vi "Read_fastseq.vi"(2 "Sequence size":u64, 5 "Readout parameters":T1(array[cluster])) -> (0 "measures":sgl[][](array[numeric]), 1 "Readout parameters out":T1(array[cluster]))   [LabVIEW 2013]
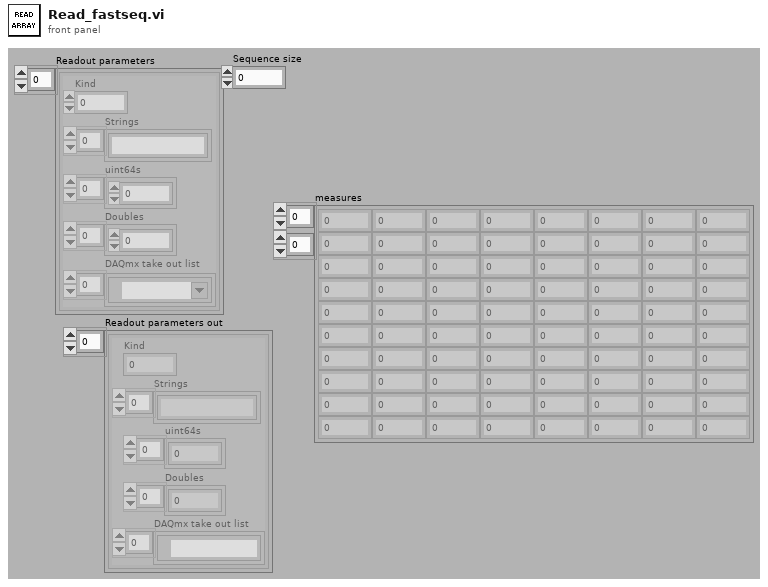
[diagram p1: front panel]
types:
  T1 = cluster{"Kind":u16, "Strings":string[], "uint64s":u64[], "Doubles":dbl[], "DAQmx take out list":refnum<k21>[]}[]
  T2 = cluster{"Kind":u16, "Strings":string[], "uint64s":u64[], "Doubles":dbl[], "DAQmx take out list":refnum<k21>[]}
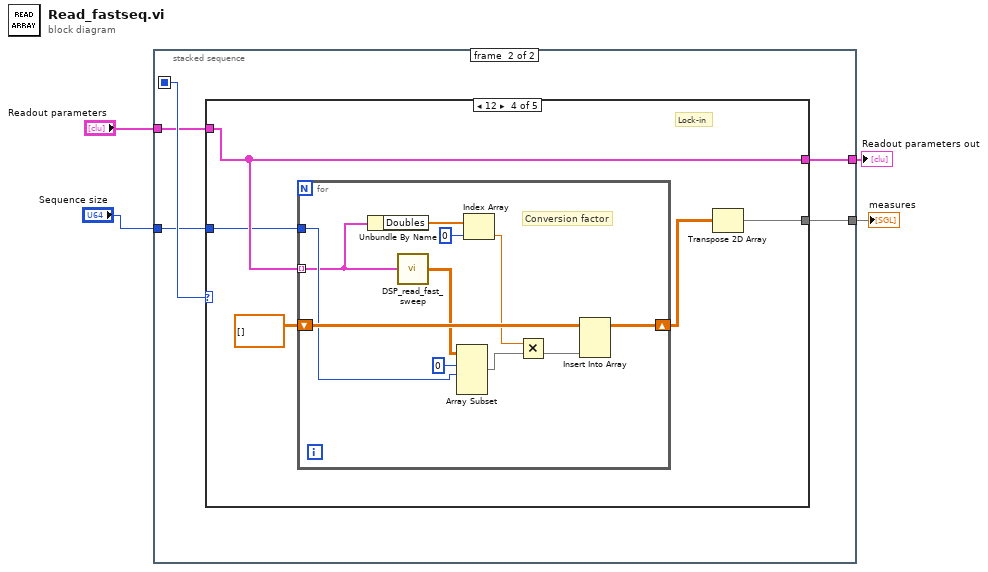
[diagram p0: block diagram]
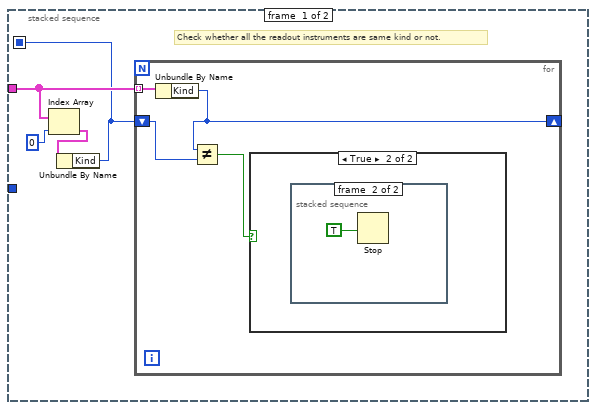
[diagram p2: hidden frame]
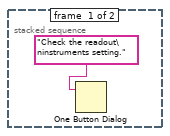
[diagram p4: hidden frame]
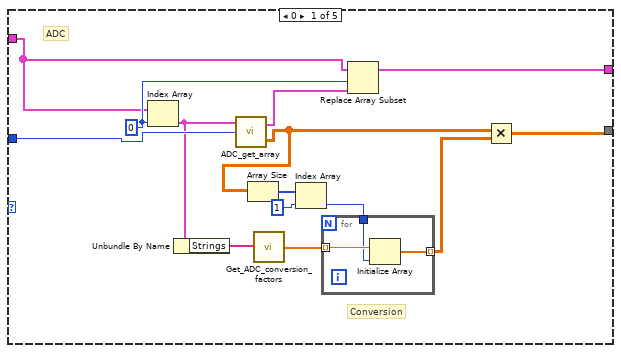
[diagram p5: hidden frame]
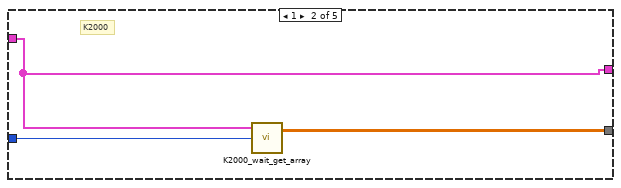
[diagram p6: hidden frame]
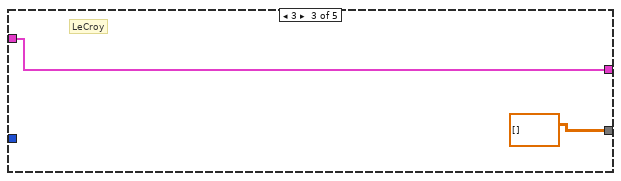
[diagram p7: hidden frame]
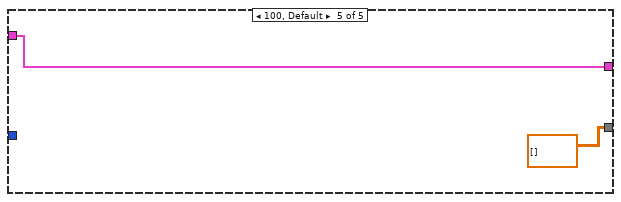
[diagram p8: hidden frame]
diagram:
  n1 = stacked-sequence {
    seq-local: [w5 _] -> [_ w19]
    tunnel: "Readout parameters" -> [w8 w18]
    tunnel: "Sequence size" -> [_ w17]
    tunnel: [_ w16] -> w2
    tunnel: [_ w15] -> w1
    frame #0 {
      # "Check whether all the readout instruments are same kind or not."
      n2 = Index Array(array=w8, index=0) -> (element=w6:T2)
      n3 = Unbundle By Name(w6) -> ("Kind"=w5:u16)
      n4 = for {
        tunnel: w8 -> [w12] mode=indexing
        shift-right: [w11] -> _
        shift-left: w5 -> [w10]
        n5 = Unbundle By Name(w12) -> ("Kind"=w11:u16)
        n6 = Not Equal?(x=w11, y=w10) -> (x != y?=w9:bool)
        n7 = case shown="True" w9 {
          frame False {
          }
          frame True {
            n8 = stacked-sequence {
              frame #0 {
                n9 = One Button Dialog(message="Check the readout\ninstruments setting.") -> ()  [unwired: 1 in, 1 out]
              }
              frame #1 {
                n10 = Stop(stop? (T)=TRUE) -> ()
              }
            }
          }
        }
      }
    }
    frame #1 {
      n11 = case shown="12" w19 {
        tunnel: w18 -> [w31 w37 w40 w46 w58]
        tunnel: w17 -> [w33 w39 _ w45 _]
        tunnel: [w22 w38 sgl[][] [] w42 sgl[][] []] -> w16
        tunnel: [w29 w37 w40 w46 w58] -> w15
        frame 0 {
          w32 = 0
          # "Conversion"
          # "ADC"
          n12 = Index Array(array=w31, index=w32) -> (element=w28:T2)
          n13 = Unbundle By Name(w28) -> ("Strings"=w27:string[])
          n14 = call "ADC_get_array.vi"("Fast sequence size"=w33, "Inst_parameter"=w28) -> ("measures"=w21:sgl[][], "Inst_parameter out"=w30:T2)  [unwired: 1 in]
          n15 = Array Size(array=w21) -> (size(s)=w25:i32[])
          n16 = call "Get_ADC_conversion_factors.vi"("Strings"=w27) -> ("Conversion factors"=w26:dbl[])
          n17 = Index Array(array=w25, index=1) -> (element=w23:i32)
          n18 = for {
            tunnel: w26 -> [w36] mode=indexing
            tunnel: w23 -> [w35]
            tunnel: [w34] -> w20 mode=indexing
            n19 = Initialize Array(w36, w35) -> (w34:dbl[])
          }
          n20 = Replace Array Subset(array=w31, new element=w30, index=w32) -> (w29:T1)
          n21 = Multiply(x=w21, y=w20) -> (x*y=w22:dbl[][])
        }
        frame 1 {
          # "K2000"
          n22 = call "K2000_wait_get_array.vi"("samples"=w39, "Readout parameters"=w37) -> ("measures"=w38:sgl[][])  [unwired: 1 in, 1 out]
        }
        frame 3 {
          # "LeCroy"
        }
        frame 12 {
          # "Lock-in"
          n23 = for {
            tunnel: w46 -> [w52] mode=indexing
            tunnel: w45 -> [w53]
            shift-right: [w49] -> w43
            shift-left: sgl[][] [] -> [w57]
            # "Conversion factor"
            n24 = Unbundle By Name(w52) -> ("Doubles"=w51:dbl[])
            n25 = call "DSP_read_fast_sweep.vi"("inst param"=w52) -> ("Data"=w56:dbl[][])
            n26 = Array Subset(array=w56, index (row)=0, length (row)=w53) -> (w54:dbl[][])  [unwired: 2 in]
            n27 = Index Array(array=w51, index=0) -> (element=w47:dbl)
            n28 = Multiply(x=w47, y=w54) -> (x*y=w48:dbl[][])
            n29 = Insert Into Array(array=w57, new element=w48) -> (w49:sgl[][])  [unwired: 2 in]
          }
          n30 = Transpose 2D Array(2D array=w43) -> (transposed array=w42:sgl[][])
        }
        frame 100, Default {
        }
      }
    }
  }
  "measures" <- w2
  "Readout parameters out" <- w1
